vi "Retry Dialog.vi"(6 "Limit Status":T1, 8 "error in":errorcluster, 9 "Data String":string[][](array[string]), 10 "Col Header String":string[](array[string])) -> (0 "error out":errorcluster, 2 "Next Action":enum16{"Retry", "Ignore", "Abort"}(ring))   [LabVIEW 2020, in "GUCalibration2.lvlib"]
uses:
  GUCalibration2.lvlib
  <vilib>/Utility/miscctls.llb/LVRowAndColumnUnsignedTypeDef.ctl
panel:
  in  "Abort":bool
  in  "Ignore":bool
  in  "Retry":bool
  out "Result Table":string[][](table)
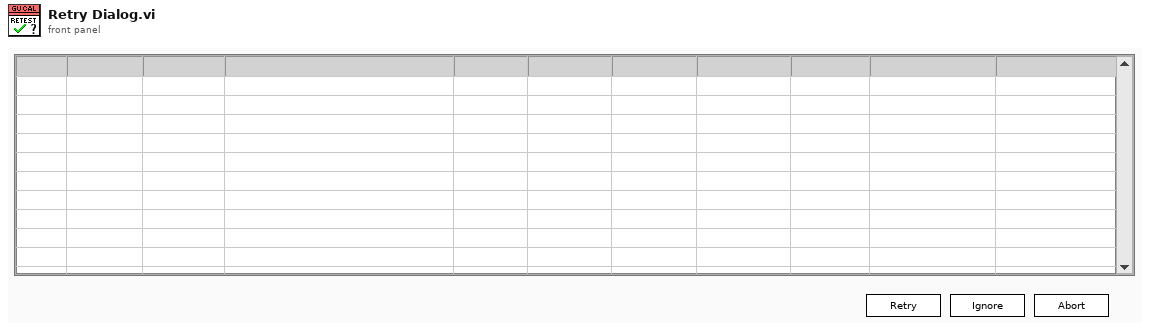
[diagram p1: front panel]
types:
  T1 = cluster{"Check Limit":bool[], "Cal Limit":bool[], "Cal GU Pass":bool[][], "Check GU Pass":bool[][], "Site Num":i32[], "GU Num":string[][]}
  T2 = typedef "LVRowAndColumnUnsignedTypeDef.ctl" = cluster{"Row":u32, "Column":u32}
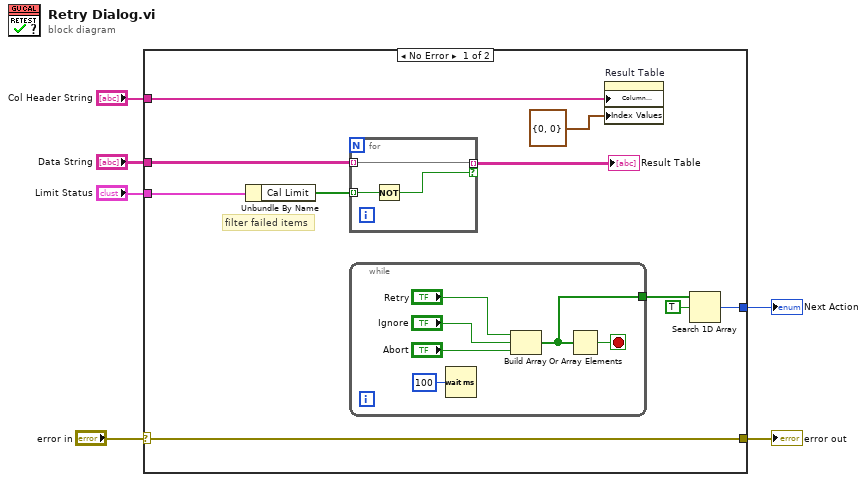
[diagram p0: block diagram]
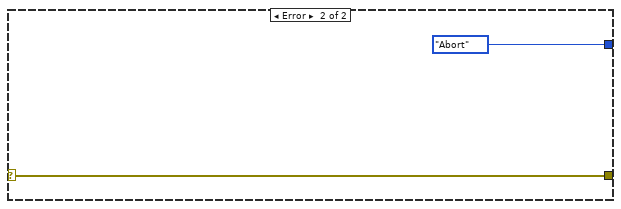
[diagram p2: hidden frame]
diagram:
  n1 = case shown="No Error" "error in" {
    selector: "error in" -> [w15 w27]
    tunnel: [w15 w27] -> w5
    tunnel: [w12 enum16{"Retry", "Ignore", "Abort"}."Abort" ("Next Action 2")] -> w4
    tunnel: "Limit Status" -> [w11 _]
    tunnel: "Col Header String" -> [w8 _]
    tunnel: "Data String" -> [w9 _]
    frame No Error {
      # "filter failed items"
      n2 = Unbundle By Name(w11) -> ("Cal Limit"=w10:bool[])
      n3 = for {
        tunnel: w10 -> [w18] mode=indexing
        tunnel: w9 -> [w19] mode=indexing
        tunnel: [w19] -> w7 mode=indexing if=w17
        n4 = Not(x=w18) -> (.not. x?=w17:bool)
      }
      "Result Table" <- w7
      n5 = while {
        tunnel: [w20] -> w14
        stop <- w21 stop-if-true
        n6 = Wait (ms)(milliseconds to wait=u32 100) -> ()  [unwired: 1 out]
        n7 = Build Array("Retry", "Ignore", "Abort") -> (w20:bool[])
        n8 = Or Array Elements(Boolean array=w20) -> (logical OR=w21:bool)
      }
      n9 = property on="Result Table" class="Tbl (strict)"("Column Headers[]"=w8, "Index Values"=T2 {"Row"=0, "Column"=0}) -> ()  [unwired: 2 in, 2 out]
      n10 = Search 1D Array(1D array=w14, element=TRUE) -> (index of element=w12:i32)  [unwired: 1 in]
    }
    frame Error {
    }
  }
  "error out" <- w5
  "Next Action" <- w4
